vi "Error stream reader global.vi"() -> ()   [LabVIEW 2015]
panel:
  in  "Error stream reader":refnum<k21>
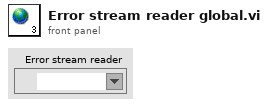
[diagram p1: front panel]
diagram:
